vi "WriteConfigure__slk_mt.vi"(8 "error in (no error)":errorcluster, 10 "configure values":string[][](array[string]), 11 "refnum in":T1) -> (0 "error out":errorcluster, 3 "refnum out":T1)   [LabVIEW 2010, in "Lazyboots Menu Tool.lvlib"]
doc: "Sets the values to the configure file.\n\n<b>Values:</b>\n[ [Section, Key, Value], [Section, Key, Value], ..., [Section, Key, Value] ]"
uses:
  Library/Lazyboots Menu Tool.lvlib
  <vilib>/Utility/config.llb/Config Data RefNum.ctl
  <vilib>/Utility/config.llb/Write Key (String).vi
  <vilib>/Utility/config.llb/NI_LVConfig.lvlib
panel:
  # "WriteConfigure__slk_mt.vi\nSets the values to the configure file.\n\nNOTICE -- YOU MUST LEAVE THIS NOTICE IN PLACE.\n\nCopyright (c) 2011, LIANG LIU Shawn.Liu.cn@gmail.com\nAll rights reserved.\n\nRedistribution and use in source and binary forms, with or without modification, are permitted provided that the following conditions are met:\n-Redistributions of source code must retain the above copyright notice, this list of conditions and the following disclaimer.\n-Redistributions in binary form must reproduce the above copyright notice, this list of conditions and the following disclaimer in the documentation and/or other materials provided with the distribution.\n-Neither the name of the eLp nor the names of its contributors may be used to endorse or promote products derived from this software without specific prior written permission.\n\nTHIS SOFTWARE IS PROVIDED BY THE COPYRIGHT HOLDERS AND CONTRIBUTORS \"AS IS\" AND ANY EXPRESS OR IMPLIED WARRANTIES, INCLUDING, BUT NOT LIMITED TO, THE IMPLIED WARRANTIES OF MERCHANTABILITY AND FITNESS FOR A PARTICULAR PURPOSE ARE DISCLAIMED. IN NO EVENT SHALL THE COPYRIGHT HOLDER OR CONTRIBUTORS BE LIABLE FOR ANY DIRECT, INDIRECT, INCIDENTAL, SPECIAL, EXEMPLARY, OR CONSEQUENTIAL DAMAGES (INCLUDING, BUT NOT LIMITED TO, PROCUREMENT OF SUBSTITUTE GOODS OR SERVICES; LOSS OF USE, DATA, OR PROFITS; OR BUSINESS INTERRUPTION) HOWEVER CAUSED AND ON ANY THEORY OF LIABILITY, WHETHER IN CONTRACT, STRICT LIABILITY, OR TORT (INCLUDING NEGLIGENCE OR OTHERWISE) ARISING IN ANY WAY OUT OF THE USE OF THIS SOFTWARE, EVEN IF ADVISED OF THE POSSIBILITY OF SUCH DAMAGE."
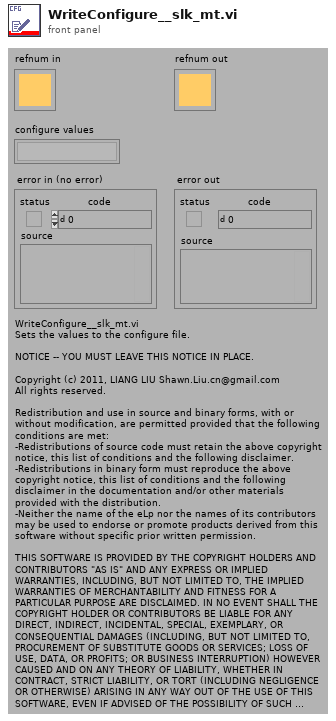
[diagram p1: front panel]
types:
  T1 = typedef "NI_LVConfig.lvlib/Config Data RefNum.ctl" = refnum<k1>
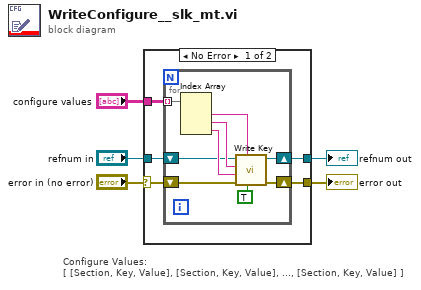
[diagram p0: block diagram]
diagram:
  # "Configure Values:\n[ [Section, Key, Value], [Section, Key, Value], ..., [Section, Key, Value] ]"
  n1 = case shown="No Error" "error in (no error)" {
    selector: "error in (no error)" -> [w8 w21]
    tunnel: "configure values" -> [w10 _]
    tunnel: "refnum in" -> [w9 w20]
    tunnel: [w7 w21] -> w2
    tunnel: [w6 w20] -> w1
    frame No Error {
      n2 = for {
        tunnel: w10 -> [w19] mode=indexing
        shift-right: [w11] -> w6
        shift-left: w9 -> [w14]
        shift-right: [w13] -> w7
        shift-left: w8 -> [w12]
        n3 = Index Array(array=w19) -> (element #1=w18:string, element #2=w17:string, element #3=w15:string)  [unwired: 3 in]
        n4 = call-poly <vilib>:"Write Key.vi"("write raw string? (F)"=TRUE, "section"=w18, "error in (no error)"=w12, "value"=w15, "key"=w17, "refnum"=w14) -> ("error out"=w13:errorcluster, "refnum out"=w11:T1)  [unwired: 4 out]
      }
    }
    frame Error {
    }
  }
  "error out" <- w2
  "refnum out" <- w1
